vi "Get Channel Properties.vi"() -> ()   [LabVIEW 2017]
uses:
  <vilib>/SLSC/Initialize Session with Devices.vi
  <vilib>/SLSC/Get Phys Chan Property (Bool).vi
  <vilib>/SLSC/Get Phys Chan Property (I32).vi
  <vilib>/SLSC/Close Session.vi
  <vilib>/SLSC/SLSC.lvlib
panel:
  out "State.Load":i32[](array[numeric])
  out "Channel names":string[](array[string])
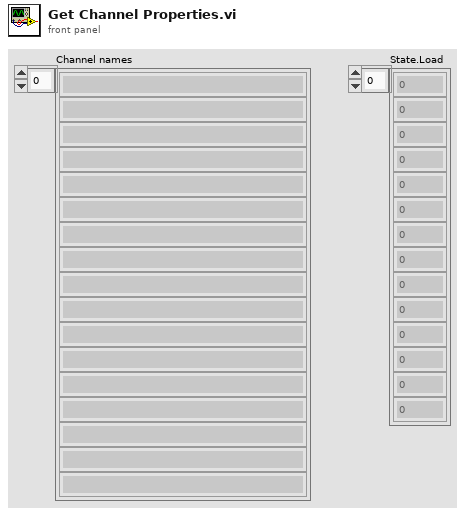
[diagram p1: front panel]
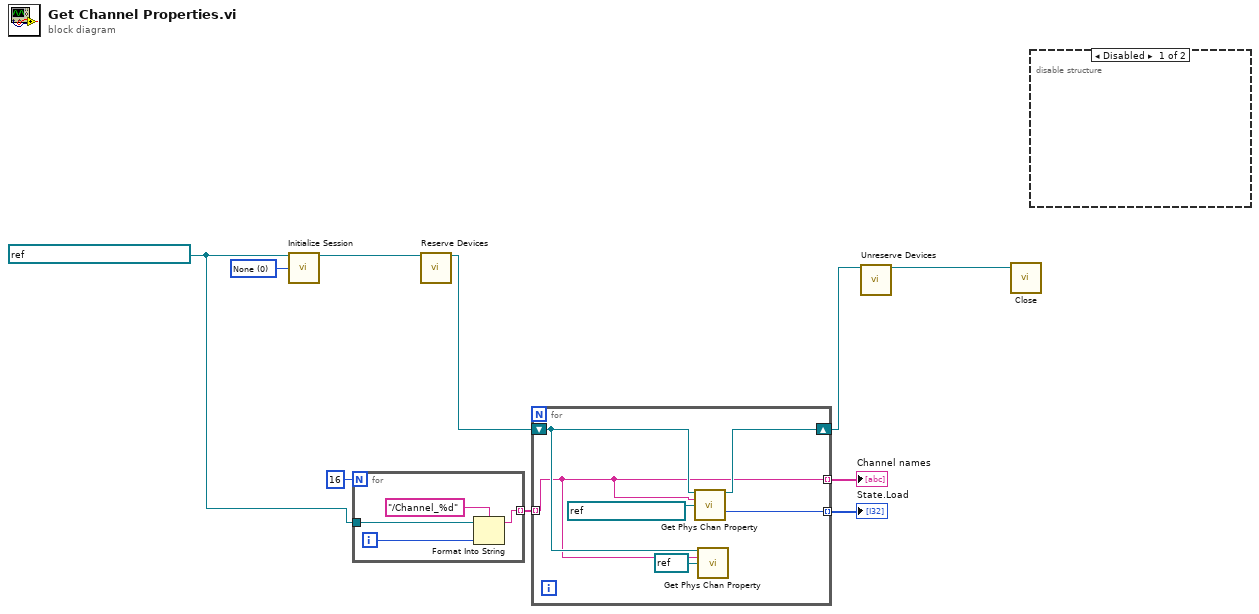
[diagram p0: block diagram]
diagram:
  w10 = 0 items=["None"=0, "Read Only"=1, "Read/Write"=3] ("reservation access (Read/Write)")
  w2 = refnum<k21> "SLSC-12001-0317E1AA-Mod2" ("devices")
  n1 = call-poly <vilib>:"Initialize Session.vi"("devices"=w2, "reservation access (Read/Write)"=w10) -> ("session out"=w8:refnum<k21>)  [unwired: 12 in, 1 out]
  n2 = for {
    N: 16 -> [_]
    tunnel: w2 -> [w12]
    tunnel: [w11] -> w5 mode=indexing
    i -> [w13]
    n3 = Format Into String(format string="/Channel_%d", initial string=w12, w13) -> (resulting string=w11:string)  [unwired: 1 in, 1 out]
  }
  n4 = call <vilib>:"Reserve Devices.vi"("session in"=w8) -> ("session out"=w6:refnum<k21>)  [unwired: 13 in, 1 out]
  n5 = for {
    tunnel: w5 -> [w16] mode=indexing
    tunnel: [w19] -> w3 mode=indexing
    tunnel: [w16] -> w4 mode=indexing
    shift-right: [w18] -> w1
    shift-left: w6 -> [w17]
    n6 = call-poly <vilib>:"Get Phys Chan Property.vi"("session in"=w17, "physical channels"=w16, "property"=refnum<k21> "NI.FIU.State.Load") -> ("session out"=w18:refnum<k21>, "property value"=w19:i32)  [unwired: 10 in, 1 out]
    n7 = call-poly <vilib>:"Get Phys Chan Property.vi"("session in"=w17, "physical channels"=w16, "property"=refnum<k21> refnum) -> ()  [unwired: 10 in, 3 out]
  }
  "Channel names" <- w4
  "State.Load" <- w3
  n8 = call <vilib>:"Unreserve Devices.vi"("session in"=w1) -> ("session out"=w7:refnum<k21>)  [unwired: 13 in, 1 out]
  n9 = call-poly <vilib>:"Close.vi"("session in"=w7) -> ()  [unwired: 14 in, 1 out]
  n10 = disable-structure shown="Disabled" {
    frame Disabled {
    }
    frame Enabled {
    }
  }
